vi "EventClient_UnsubscribeEvents.vi"(8 "error in (no error)":errorcluster, 10 "Events":string[](array[string]), 11 "reference":T1) -> (0 "error out":errorcluster, 3 "reference out":T1)   [LabVIEW 2018]
uses:
  EventClient_ObjectReference.ctl
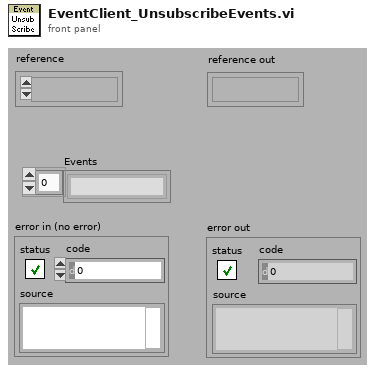
[diagram p1: front panel]
types:
  T1 = typedef "EventClient_ObjectReference.ctl" = refnum<k1>
  T2 = cluster{"Client":refnum<queue>, "Sub Events":string[], "PrvData":variant, "MyName":string}
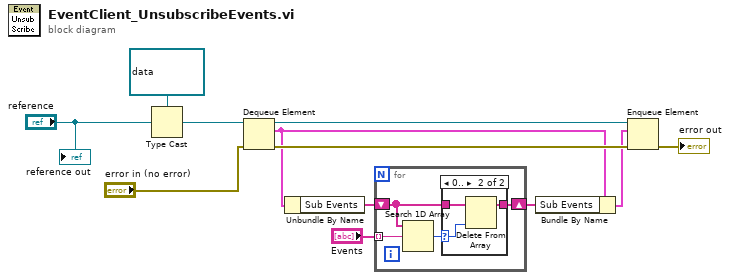
[diagram p0: block diagram]
diagram:
  n1 = Type Cast(type=refnum<queue> refnum ("queue out"), x="reference") -> (*(type *) &x=w11:refnum<queue>)
  n2 = Dequeue Element(queue=w11, error in (no error)="error in (no error)") -> (queue out=w10:refnum<queue>, element=w8:T2, error out=w9:errorcluster)  [unwired: 2 out]
  n3 = Unbundle By Name(w8) -> ("Sub Events"=w5:string[])
  n4 = for {
    shift-right: [w14] -> w6
    shift-left: w5 -> [w13]
    tunnel: "Events" -> [w16] mode=indexing
    n5 = Search 1D Array(1D array=w13, element=w16) -> (index of element=w15:i32)  [unwired: 1 out]
    n6 = case shown="0.." w15 {
      selector: w15 -> [_ w18]
      tunnel: [w17 w19] -> w14
      tunnel: w13 -> [w17 w20]
      frame ..-1 {
      }
      frame 0.. {
        n7 = Delete From Array(array=w20, index=w18) -> (array with subset deleted=w19:string[])  [unwired: 1 in, 1 out]
      }
    }
  }
  n8 = Bundle By Name(cluster=w8, "Sub Events"=w6) -> (w7:T2)
  n9 = Enqueue Element(queue=w10, element=w7, error in (no error)=w9) -> (error out=→"error out":errorcluster)  [unwired: 3 out]
  "reference out" <- "reference"
